vi "Channel_reviser.vi"(11 "CHANNEL_ARRAY":i64[](array[numeric])) -> (3 "CHANNEL_ARRAY_revised":i64[](array[numeric]))   [LabVIEW 2014]
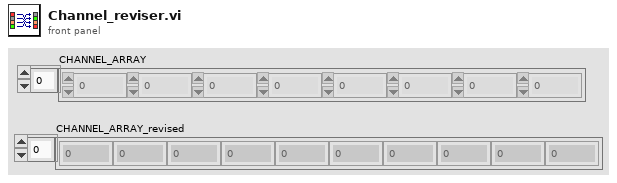
[diagram p1: front panel]
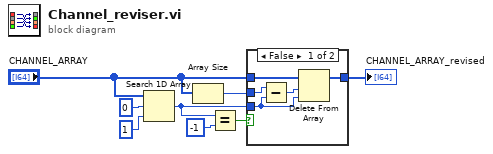
[diagram p0: block diagram]
diagram:
  n1 = Search 1D Array(1D array="CHANNEL_ARRAY", element=i64 0, start index (0)=1) -> (index of element=w2:i32)
  n2 = Array Size(array="CHANNEL_ARRAY") -> (size(s)=w3:i32)
  n3 = Equal?(x=w2, y=-1) -> (x = y?=w5:bool)
  n4 = case shown="False" w5 {
    tunnel: "CHANNEL_ARRAY" -> [w13 w14]
    tunnel: [w12 w14] -> w1
    tunnel: w3 -> [w11 _]
    tunnel: w2 -> [w9 _]
    frame False {
      n5 = Subtract(x=w11, y=w9) -> (x-y=w10:i32)
      n6 = Delete From Array(array=w13, length=w10, index=w9) -> (array with subset deleted=w12:i64[])  [unwired: 1 out]
    }
    frame True {
    }
  }
  "CHANNEL_ARRAY_revised" <- w1
